vi "SIM Calculate Machine Epsilon.vi"() -> (0 "min float":dbl, 1 "machine eps":dbl)   [LabVIEW 2014]
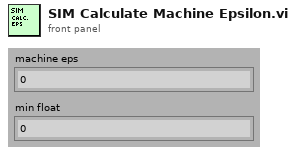
[diagram p1: front panel]
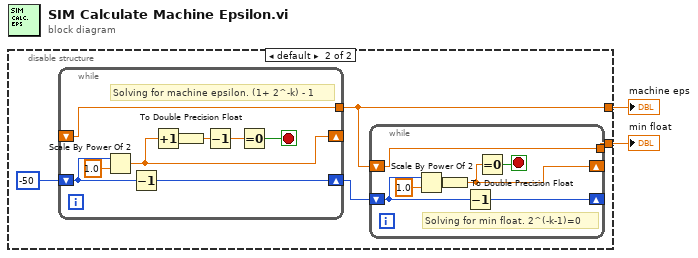
[diagram p0: block diagram]
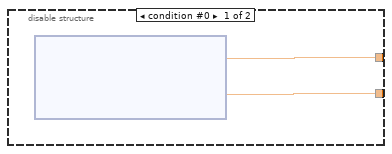
[diagram p2: hidden frame]
diagram:
  n1 = disable-structure shown="default" {
    disable-tunnel: [w4 w6] -> w2
    disable-tunnel: [w3 w5] -> w1
    frame condition #0 {
      n2 = node() -> (w4:dbl, w3:dbl)
    }
    frame condition #1 (active) {
      n3 = while {
        shift-right: [w21] -> w8
        shift-left: -50 -> [w18]
        shift-right: [w17] -> _
        shift-left: _ -> [w20]
        tunnel: [w20] -> w6
        stop <- w24 stop-if-true
        # "Solving for machine epsilon. (1+ 2^-k) - 1"
        n4 = Scale By Power Of 2(n=w18, x=1.0) -> (x*2^n=w17:dbl)
        n5 = Decrement(x=w18) -> (x-1=w21:i32)
        n6 = Increment(x=w17) -> (x+1=w23:dbl)
        n7 = To Double Precision Float(number=w23) -> (double precision float=w16:dbl)
        n8 = Decrement(x=w16) -> (x-1=w22:dbl)
        n9 = Equal To 0?(x=w22) -> (x = 0?=w24:bool)
      }
      n10 = while {
        shift-right: [w12] -> _
        shift-left: w8 -> [w13]
        shift-right: [w9] -> _
        shift-left: w6 -> [w15]
        tunnel: [w15] -> w5
        stop <- w11 stop-if-true
        # "Solving for min float. 2^(-k-1)=0"
        n11 = Scale By Power Of 2(n=w13, x=1.0) -> (x*2^n=w10:dbl)
        n12 = To Double Precision Float(number=w10) -> (double precision float=w9:dbl)
        n13 = Decrement(x=w13) -> (x-1=w12:i32)
        n14 = Equal To 0?(x=w9) -> (x = 0?=w11:bool)
      }
    }
  }
  "machine eps" <- w2
  "min float" <- w1
